vi "Olej srednia.vi"() -> ()   [LabVIEW 2017, in "GUI.lvlib"]
uses:
  Libraries/GUI/GUI.lvlib
panel:
  out "Gauge":dbl(knob) scale=0.0..10.0
  # "Temperatura"
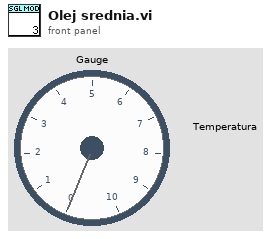
[diagram p1: front panel]
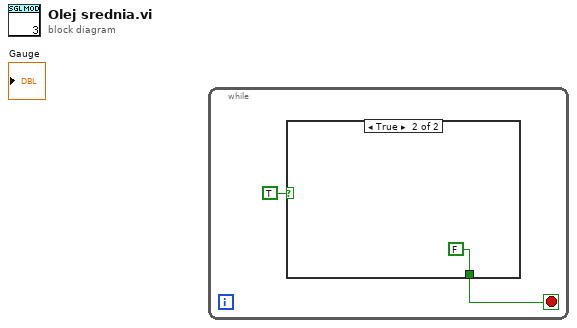
[diagram p0: block diagram]
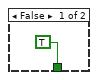
[diagram p2: hidden frame]
diagram:
  n1 = while {
    stop <- w2 stop-if-true
    n2 = case shown="True" TRUE {
      tunnel: [TRUE FALSE] -> w2
      frame False {
      }
      frame True {
      }
    }
  }
